vi "PSTR-Restore Spont PSD.vi"(0 "WaveformGraph in":refnum<vi>, 5 "Data":T1, 11 "error in (no error)":errorcluster) -> (15 "error out":errorcluster)   [LabVIEW 2020]
uses:
  Typedefs/PSTR-Data.ctl
  Typedefs/PSTR-Model Fit.ctl
  Typedefs/PSTR-Fit Parameters.ctl
  epl-vi-lib/Utility VIs/Conversion VIs/Create Waveform Cluster (1D).vi
panel:
  # "NF x NL x 2 x Npts"
  # "NF x NL x Npts"
  # "NF x NL"
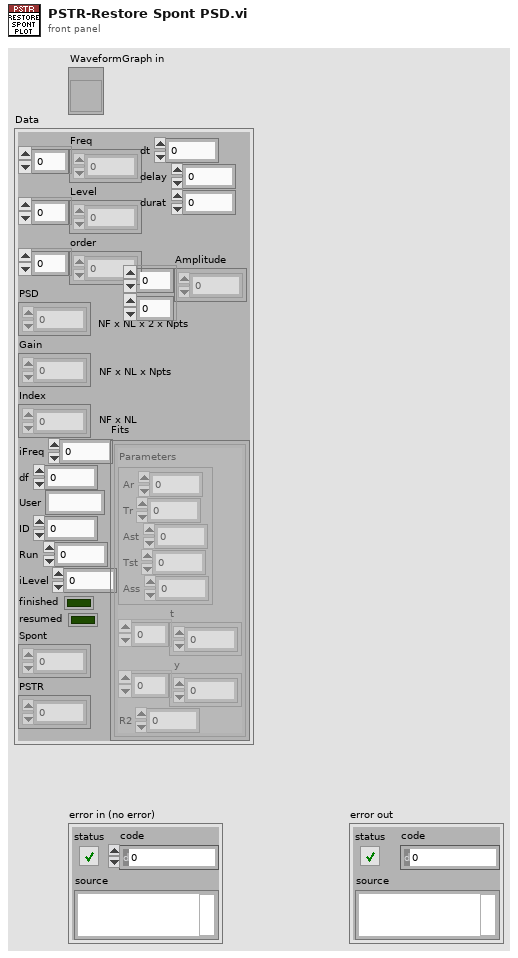
[diagram p1: front panel]
types:
  T1 = typedef "PSTR-Data.ctl" = cluster{"Freq":dbl[], "Level":dbl[], "order":i32[], "PSD":dbl[][][][], "Gain":dbl[][][], "Index":dbl[][], "iFreq":i32, "df":dbl, "User":string, "ID":i32, "Run":i32, "iLevel":i32, "finished":bool, "resumed":bool, "Spont":dbl[][], "PSTR":dbl[][][], "dt":dbl, "delay":dbl, "durat":dbl, "Fits":T2[][], "Amplitude":dbl[][]}
  T2 = typedef "PSTR-Model Fit.ctl" = cluster{"Parameters":T3, "t":dbl[], "y":dbl[], "R2":dbl}
  T3 = typedef "PSTR-Fit Parameters.ctl" = cluster{"Ar":dbl, "Tr":dbl, "Ast":dbl, "Tst":dbl, "Ass":dbl}
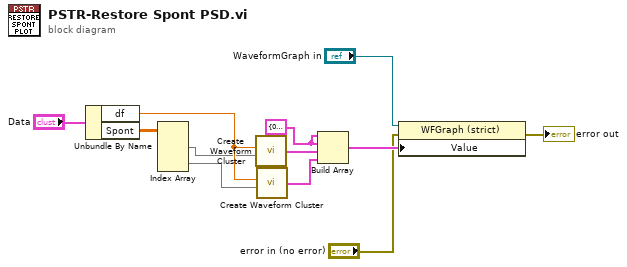
[diagram p0: block diagram]
diagram:
  w3 = cluster{dbl, "dx":dbl, "Y":dbl[]} {0.0, "dx"=0.0, "Y"=[]} ("waveform cluster")
  n1 = Unbundle By Name("Data") -> ("df"=w10:dbl, "Spont"=w11:dbl[][])
  n2 = Index Array(array=w11) -> (element #1=w2:dbl[], element #2=w1:dbl[])  [unwired: 4 in]
  n3 = call-poly "Create Waveform Cluster.vi"("dx"=w10, "Y"=w2) -> ("waveform cluster"=w5:cluster{dbl, "dx":dbl, "Y":dbl[]})  [unwired: 3 in]
  n4 = call-poly "Create Waveform Cluster.vi"("dx"=w10, "Y"=w1) -> ("waveform cluster"=w4:cluster{dbl, "dx":dbl, "Y":dbl[]})  [unwired: 3 in]
  n5 = Build Array(w3, w3, w5, w4) -> (w9:cluster{dbl, "dx":dbl, "Y":dbl[]}[])
  n6 = property class="WFGraph (strict)"(reference="WaveformGraph in", error in="error in (no error)", "Value"=w9) -> (error out=→"error out":errorcluster)  [unwired: 1 out]
